vi "VCS Set Object_UINT8.vi"(0 "axis In":cluster{"keyHandle":u32, "nodeId":u16}={"keyHandle"=0, "nodeId"=1}, 5 "object in":T1 {"object subIndex" format="%x"; "object index" format="%x"}, 11 "error in (no error)":errorcluster) -> (4 "axis Out":cluster{"keyHandle":u32, "nodeId":u16}={"keyHandle"=0, "nodeId"=1}, 15 "error out":errorcluster)   [LabVIEW 2010]
doc: "<B>VCS Set Object</B> writes an UINT8 object value at the given index and sub index from object dictionary."
uses:
  Resources/EposCmd.dll
  Resources/EposCmd64.dll
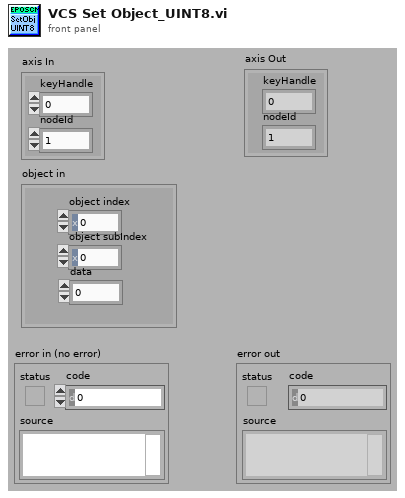
[diagram p1: front panel]
types:
  T1 = cluster{"object index":u16, "object subIndex":u8, "data":u8}
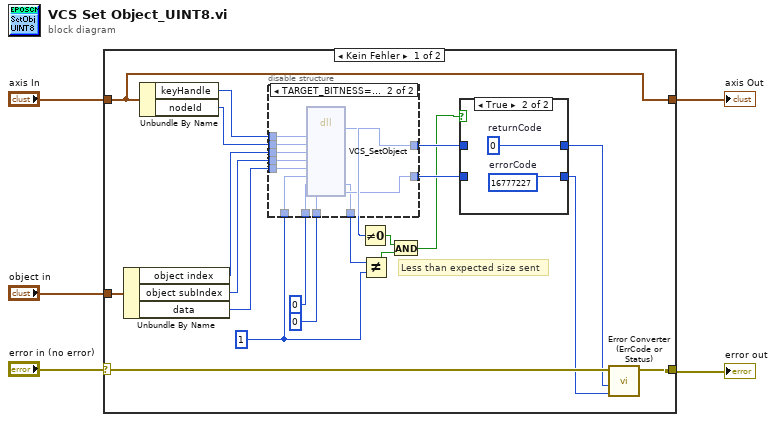
[diagram p0: block diagram]
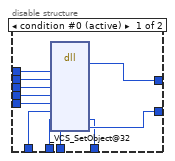
[diagram p2: hidden frame]
diagram:
  n1 = case shown="Kein Fehler" "error in (no error)" {
    selector: "error in (no error)" -> [w8 w53]
    tunnel: [w9 w53] -> w4
    tunnel: "axis In" -> [w14 w52]
    tunnel: "object in" -> [w25 _]
    tunnel: [w14 w52] -> w1
    frame No Error {
      w10 = u32 1
      # "Less than expected size sent"
      n2 = Unbundle By Name(w25) -> ("object index"=w22:u16, "object subIndex"=w21:u8, "data"=w11:u8)
      n3 = Unbundle By Name(w14) -> ("keyHandle"=w24:u32, "nodeId"=w23:u16)
      n4 = disable-structure shown="TARGET_BITNESS==64" {
        disable-tunnel: w24 -> [w36 w47]
        disable-tunnel: w23 -> [w35 w46]
        disable-tunnel: w22 -> [w34 w45]
        disable-tunnel: w21 -> [w33 w44]
        disable-tunnel: [w32 w43] -> w20
        disable-tunnel: [w31 w42] -> w19
        disable-tunnel: [w30 w41] -> w18
        disable-tunnel: u32 0 ("pNbOfBytesWritten") -> [w29 w40]
        disable-tunnel: u32 0 ("pErrorCode") -> [w28 w39]
        disable-tunnel: w11 -> [w27 w38]
        disable-tunnel: w10 -> [w26 w37]
        frame condition #0 (active) {
          n5 = dll-call lib="C:/Sources/LabView/maxon EPOS/Resources/EposCmd.*" fn="_VCS_SetObject@32"("KeyHandle"=w36, "NodeId"=w35, "ObjectIndex"=w34, "ObjectSubIndex"=w33, "Data"=w27, "NbOfBytesToWrite"=w26, "pNbOfBytesWritten"=w29, "pErrorCode"=w28) -> (w30:i32, "pNbOfBytesWritten"=w31:u32, "pErrorCode"=w32:u32)  [unwired: 9 in, 2 out]
        }
        frame condition #1 {
          n6 = dll-call lib="C:/setup/Resources/EposCmd64.*" fn="VCS_SetObject" ("EposCmd.dll:_VCS_SetObject@32")("KeyHandle"=w47, "NodeId"=w46, "ObjectIndex"=w45, "ObjectSubIndex"=w44, "Data"=w38, "NbOfBytesToWrite"=w37, "pNbOfBytesWritten"=w40, "pErrorCode"=w39) -> ("Rückgabetyp"=w41:i32, "pNbOfBytesWritten"=w42:u32, "pErrorCode"=w43:u32)  [unwired: 9 in, 2 out]
        }
      }
      n7 = Not Equal To 0?(x=w18) -> (x != 0?=w16:bool)
      n8 = Not Equal?(x=w19, y=w10) -> (x != y?=w17:bool)
      n9 = And(x=w16, y=w17) -> (x .and. y?=w15:bool)
      n10 = case shown="True" w15 {
        tunnel: [w49 w51] -> w6
        tunnel: [w48 w50] -> w7
        tunnel: w18 -> [w49 _]
        tunnel: w20 -> [w48 _]
        frame False {
        }
        frame True {
          w50 = u32 16777227  # errorCode
          w51 = 0  # returnCode
        }
      }
      n11 = call "Error Converter (ErrCode or Status).vi"("error code"=w7, "return type"=w6, "error in (no error)"=w8) -> ("error out"=w9:errorcluster)  [unwired: 7 in]
    }
    frame Error {
    }
  }
  "error out" <- w4
  "axis Out" <- w1
